vi "DSF.Engine.Memory.Buffer.Get Buffer Size.vi"(11 "Buffer in":refnum<class "DSF.Engine.Memory.Buffer.lvclass">) -> (2 "buffer size":u64, 3 "Buffer out":refnum<class "DSF.Engine.Memory.Buffer.lvclass">)   [LabVIEW 2017, in "Data Sharing Framework Engine.lvlib" / "DSF.Engine.Memory.Buffer.lvclass"]
uses:
  DSF.Engine.Memory.Buffer.lvclass
  DSF.Engine.Memory.Buffer.lvclass/DSF.Engine.Memory.Buffer.ctl
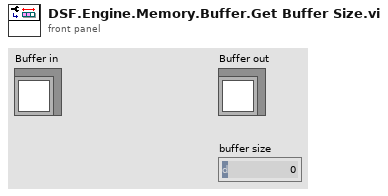
[diagram p1: front panel]
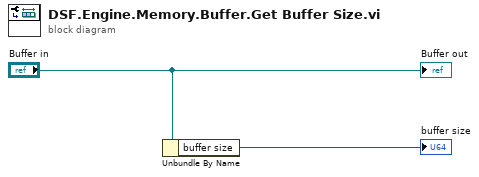
[diagram p0: block diagram]
diagram:
  n1 = Unbundle By Name("Buffer in") -> ("buffer size"=→"buffer size":u64)
  "Buffer out" <- "Buffer in"
